vi "LoopTiming.vi"() -> ()   [LabVIEW 2015]
uses:
  <vilib>/Platform/TimedLoop/XDataNode/timing_clust.ctl
  <vilib>/Platform/TimedLoop/XDataNode/nitl_modes.ctl
  <vilib>/Platform/TimedLoop/XDataNode/wakeup.ctl
  <vilib>/Platform/TimedLoop/XDataNode/XDataNode.xnode
  <vilib>/Platform/TimedLoop/XDataNode/XDNodeRunTimeDep.lvlib
  <vilib>/ptbypt/NI_PtbyPt.lvlib
panel:
  out "Target: 20ms":dbl format="%0.2f"
  out "Target: 1000us":dbl format="%0.2f"
  out "Target: 10000us":dbl format="%0.2f"
  out "Target: 10000us":dbl format="%0.2f"
  out "Interface Loop Time":i64
  out "Low Level Loop Time":u16
  out "Logger Loop Time":u16
  out "High Level Loop Time":u16
  # "Current"
  # "Max"
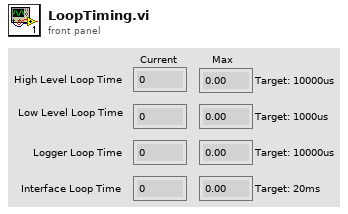
[diagram p1: front panel]
types:
  T1 = typedef "XDNodeRunTimeDep.lvlib/timing_clust.ctl" = cluster{"Expected End [f-1]":u64, "Actual End [f-1]":u64, "Finished Late? [f-1]":bool, "Expected End [i-1]":u64, "Actual End [i-1]":u64, "Finished Late? [i-1]":bool, "Expected Start [i]":u64, "Actual Start [i]":u64, "Expected Start [f]":u64, "Actual Start [f]":u64, "Source Name":string, "Structure Name":string, "Period":i64, "Deadline":i64, "Offset":i64, "Start":i64, "Priority":i32, "Timeout":i32, "Mode":T2, "Wakeup Reason":T3, "Error":errorcluster, "Source Type":string, "Secondary Source Type":string, "Global End Time":u64, "Global Start Time":u64, "Frame Duration":u64, "Iteration Duration":u64, "Assigned CPU":i32, "I/O Scan Engine Mode":u32}
  T2 = typedef "XDNodeRunTimeDep.lvlib/nitl_modes.ctl" = enum32{"No Change", "Process missed periods, maintain original phase", "Discard missed periods, maintain original phase", "Process missed periods, ignore original phase", "Discard missed periods, ignore original phase"}
  T3 = typedef "XDNodeRunTimeDep.lvlib/wakeup.ctl" = enum32{"Normal", "Aborted", "Asynchronous wakeup", "Timing source error", "Timed loop error", "Timeout"}
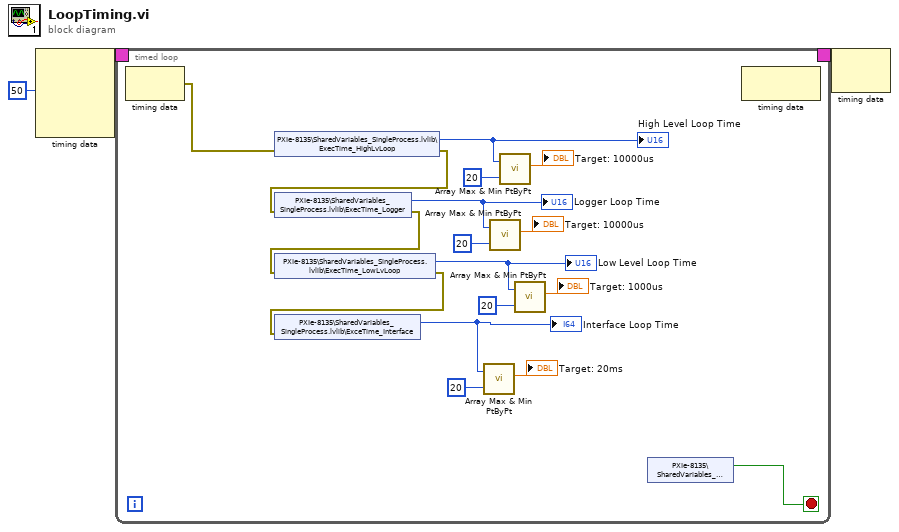
[diagram p0: block diagram]
diagram:
  n1 = node-c288(i64 50 ("Period")) -> (w3:T1)  [unwired: 3 in]
  n2 = timed-loop {
    timing: w3 -> [_]
    timing-out: [_] -> w2
    stop <- w4 stop-if-true
    n3 = node-c288() -> (w20:errorcluster)  [unwired: 1 in]
    n4 = shared-variable "PXIe-8135\\SharedVariables_SingleProcess.lvlib\\ExecTime_HighLvLoop"(error in=w20) -> (w16:u16, error out=w19:errorcluster)
    "High Level Loop Time" <- w16
    n5 = shared-variable "PXIe-8135\\SharedVariables_SingleProcess.lvlib\\ExecTime_Logger"(error in=w19) -> (w11:u16, error out=w18:errorcluster)
    "Logger Loop Time" <- w11
    n6 = shared-variable "PXIe-8135\\SharedVariables_SingleProcess.lvlib\\ExecTime_LowLvLoop"(error in=w18) -> (w8:u16, error out=w17:errorcluster)
    "Low Level Loop Time" <- w8
    n7 = shared-variable "PXIe-8135\\SharedVariables_SingleProcess.lvlib\\ExceTime_Interface"(error in=w17) -> (w5:i64)  [unwired: 1 out]
    "Interface Loop Time" <- w5
    n8 = call <vilib>:"Array Max & Min PtByPt.vi"("input data point"=w5, "sample length"=20) -> ("max value"=→"Target: 20ms":dbl)  [unwired: 1 in, 4 out]
    n9 = call <vilib>:"Array Max & Min PtByPt.vi"("input data point"=w11, "sample length"=20) -> ("max value"=→"Target: 10000us":dbl)  [unwired: 1 in, 4 out]
    n10 = call <vilib>:"Array Max & Min PtByPt.vi"("input data point"=w16, "sample length"=20) -> ("max value"=→"Target: 10000us":dbl)  [unwired: 1 in, 4 out]
    n11 = call <vilib>:"Array Max & Min PtByPt.vi"("input data point"=w8, "sample length"=20) -> ("max value"=→"Target: 1000us":dbl)  [unwired: 1 in, 4 out]
    n12 = shared-variable "PXIe-8135\\SharedVariables_Network.lvlib\\Stop RT"() -> (w4:bool)  [unwired: 1 in, 1 out]
    n13 = node-c288() -> ()  [unwired: 1 in, 1 out]
  }
  n14 = node-c288(w2) -> ()  [unwired: 1 out]
